vi "Torque, Load, and Efficiency.vi"   [LabVIEW 2014, in "NI_EP_Motor Monitoring.lvlib"]
doc: "Calculates the torque, load, and efficiency values based on the motor nameplate information. You must manually select the polymorphic instance you want to use."
uses:
  <vilib>/addons/Electrical Power/Motor Monitoring/NI_EP_Motor Monitoring.lvlib
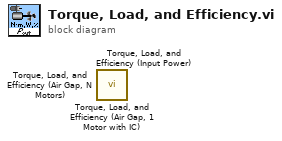
[diagram p0: block diagram]
diagram:
  n1 = call <vilib>:"Torque, Load, and Efficiency (Air Gap, 1 Motor with IC).vi"() -> ()  [unwired: 10 in, 6 out]
  n2 = call <vilib>:"Torque, Load, and Efficiency (Input Power).vi"() -> ()  [unwired: 12 in, 4 out]
  n3 = call <vilib>:"Torque, Load, and Efficiency (Air Gap, N Motors).vi"() -> ()  [unwired: 11 in, 5 out]
